vi "Shortcut Act CB.vi"(4 "Shortcut Act Data":refnum<user-event>, 5 "Event Data":T2, 6 "CtlRef":refnum<vi>, 7 "Event Common Data":cluster{"Source":T3, "Type":T4, "Time":u32} {"Source" items=["LabVIEW UI"=0, "ActiveX"=1, "User Event"=25]}) -> (0 "Discard?":bool)   [LabVIEW 2015, in "Handler UI Callbacks.lvlib"]
uses:
  Handler UI Callbacks.lvlib
  <vilib>/event_ctls.llb/eventsource.ctl
  <vilib>/event_ctls.llb/lveventtype.ctl
  <vilib>/Utility/miscctls.llb/LVPoint32TypeDef.ctl
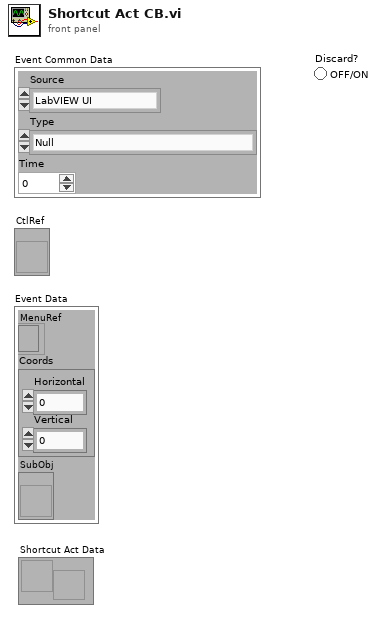
[diagram p1: front panel]
types:
  T1 = typedef "LVPoint32TypeDef.ctl" = cluster{"Horizontal":i32, "Vertical":i32}
  T2 = cluster{"MenuRef":refnum<k9>, "Coords":T1, "SubObj":refnum<vi>}
  T3 = typedef "eventsource.ctl" = u32
  T4 = typedef "lveventtype.ctl" = enum32{"Null", "Timeout", "Annotation Menu Selection", "Annotation Menu Selection?", "App Instance Close", "App Instance Close?", "Autoscale Range Change", "Bookmark Info Change", "Cell Edit", "Cell Edit?", "Cursor Grab", "Cursor Grab?", "Cursor Menu Selection", "Cursor Menu Selection?", "Cursor Move", "Cursor Release", "Data Change", "Direction Change", "Display State Change", "Drag Ended", "Drag Enter", "Drag Leave", "Drag Over", "Drag Source Update", "Drag Starting", "Drag Starting?", "Drop", "Exec State Change", "Key Down", "Key Down?", "Key Repeat", "Key Repeat?", "Key Up", "Listbox Double Click", "Menu Activation?", "Menu Selection (App)", "Menu Selection? (App)", "Menu Selection (User)", "Mouse Down", "Mouse Down?", "Mouse Enter", "Mouse Leave", "Mouse Move", "Mouse Up", "Mouse Wheel", "NI Security User Change (App)", "Pane Size", "Panel Close", "Panel Close?", "Panel Resize", "Plot Attribute Change", "Scale Range Change", "Shortcut Menu Activation?", "Shortcut Menu Selection (App)", "Shortcut Menu Selection? (App)", "Shortcut Menu Selection (User)", "Tree Double Click", "Tree Drag", "Tree Drag?", "Tree Drop", "Tree Drop?", "Tree Item Close", "Tree Item Close?", "Tree Item Open", "Tree Item Open?", "User Event", "Value Change"}
  T5 = cluster{"occurrence":refnum<k4>, "Event Data":cluster{"MenuRef":refnum<k9>, "Coords":T1, "SubObj":refnum<vi>}}
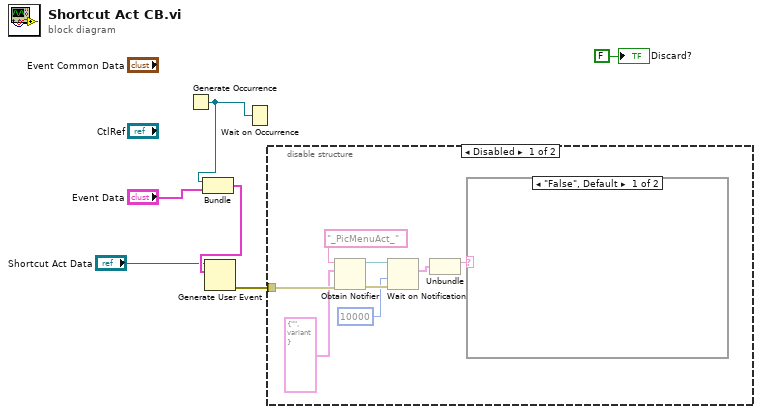
[diagram p0: block diagram]
diagram:
  n1 = Generate Occurrence() -> (w4:refnum<k4>)
  n2 = Bundle("occurrence"=w4, "Event Data"="Event Data") -> (w2:T5)  [unwired: 1 in]
  n3 = Generate User Event(user event="Shortcut Act Data", event data cluster=w2) -> (error out=w5:errorcluster)  [unwired: 2 in, 1 out]
  n4 = Wait on Occurrence(2:w4) -> ()  [unwired: 2 in, 1 out]
  n5 = disable-structure shown="Disabled" {
    disable-tunnel: w5 -> [w14 _]
    frame Disabled {
      n6 = Obtain Notifier(name (unnamed)="_PicMenuAct_", notification data type=cluster{"Cmd":string, "Data":variant} {"Cmd"="", "Data"=variant}, error in (no error)=w14) -> (notifier out=w9:refnum<notifier>, error out=w11:errorcluster)  [unwired: 1 in, 1 out]
      n7 = Wait on Notification(notifier=w9, timeout in ms (-1)=10000, error in (no error)=w11) -> (notification=w8:cluster{"Cmd":string, "Data":variant})  [unwired: 1 in, 3 out]
      n8 = Unbundle(w8) -> ("Cmd"=w7:string)  [unwired: 1 out]
      n9 = case shown="\"False\", Default" w7 {
        frame "False", Default {
        }
        frame "True" {
        }
      }
    }
    frame Enabled {
    }
  }
  "Discard?" <- FALSE ("Discard?")
